vi "FTW-Test-SQLite-OpenCloseStress.vi"() -> (0 "Test Result":errorcluster)   [LabVIEW 2014]
uses:
  src/core/database/core/FTW-SQLite-Core-DatabaseType.ctl
  src/core/database/core/FTW-SQLite-Core-PrepareStatement.vi
  src/core/error/FTW-ERR-Assert-DeveloperError.vi
  src/core/error/FTW-ERR-StatusOK.vi
  src/core/database/core/FTW-SQLite-Core-QueryDebug.vi
  src/core/time/FTW-Time-Uptime.vi
  lib/FTW-LibraryFilepath.vi
  src/core/error/FTW-ERR-ThrowError.vi
  src/core/error/FTW-ERR-ThrowGenericError.vi
  src/core/error/FTW-ERR-CallChain.vi
  src/core/string/FTW-STR-ReplaceWhitespace.vi
  src/core/database/core/FTW-SQLite-Core-LibraryReturnValue.vi
  src/core/database/FTW-SQLite-Fetch/FTW-SQLite-Fetch.xnode
  src/core/database/core/FTW-SQLite-Core-Structure.ctl
panel:
  out "Result Set":T1(array[cluster])
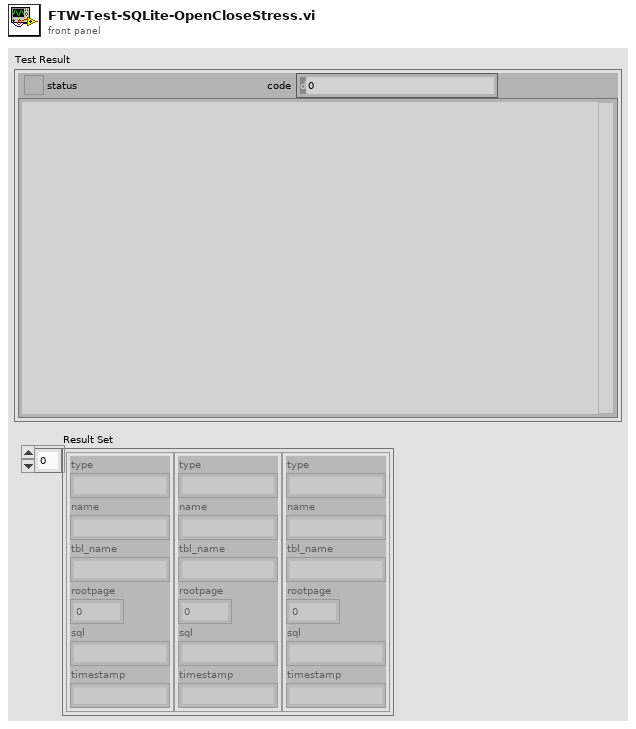
[diagram p1: front panel]
types:
  T1 = cluster{"type":string, "name":string, "tbl_name":string, "rootpage":i64, "sql":string, "timestamp":string}[]
  T2 = typedef "FTW-SQLite-Core-DatabaseType.ctl" = enum16{"Disk", "Memory"}
  T3 = cluster{"type":string, "name":string, "tbl_name":string, "rootpage":i64, "sql":string, "timestamp":string}
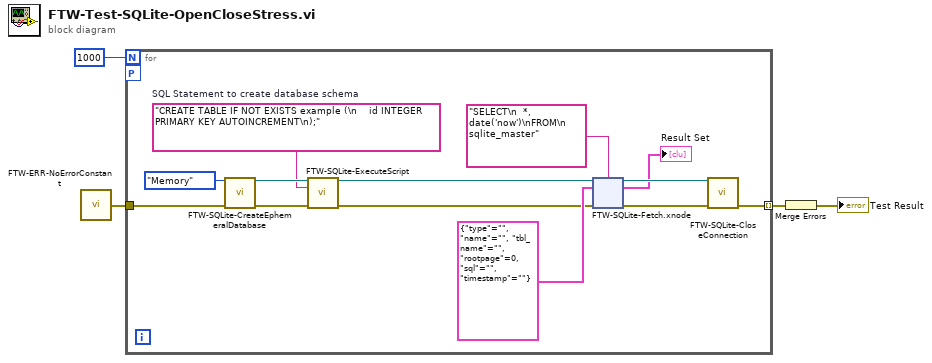
[diagram p0: block diagram]
diagram:
  n1 = call "FTW-ERR-NoErrorConstant.vi"() -> ("no error"=w1:errorcluster)
  n2 = for {
    N: 1000 -> [_]
    tunnel: [w13] -> w4 mode=indexing
    workers-P: _ -> [_]
    tunnel: w1 -> [w5]
    w15 = "CREATE TABLE IF NOT EXISTS example (\n    id INTEGER PRIMARY KEY AUTOINCREMENT\n);"  # SQL Statement to create database schema
    n3 = call "FTW-SQLite-CreateEphemeralDatabase.vi"("Database Type"=FTW-SQLite-Core-DatabaseType."Memory", "error in"=w5) -> ("SQLite Connection"=w16:refnum<data-value>, "error out"=w17:errorcluster)  [unwired: 12 in]
    n4 = call "FTW-SQLite-ExecuteScript.vi"("SQLite Connection"=w16, "SQL Script"=w15, "error in"=w17) -> ("SQLite Connection out"=w8:refnum<data-value>, "error out"=w7:errorcluster)  [unwired: 10 in, 1 out]
    n5 = xnode "FTW-SQLite-Fetch.xnode"("SQLite Connection"=w8, "SQL Script"="SELECT\n  *, date('now')\nFROM\n  sqlite_master", "Row Datatype"=T3 {"type"="", "name"="", "tbl_name"="", "rootpage"=0, "sql"="", "timestamp"=""}, "error in"=w7) -> ("SQLite Connection out"=w11:refnum<data-value>, "Result Set"=→"Result Set":T1, "error out"=w10:errorcluster)  [unwired: 1 out]
    n6 = call "FTW-SQLite-CloseConnection.vi"("SQLite Connection"=w11, "error in"=w10) -> ("error out"=w13:errorcluster)  [unwired: 13 in]
  }
  n7 = Merge Errors(w4) -> (→"Test Result":errorcluster)
